vi "Disabled - Get File Names (SubVI).vi"(4 "Alliance Color Input":string, 5 "Reload File Names":bool, 6 "Running on Robot":bool=TRUE, 7 "Robot Path":string="/c/tmp/auton/", 8 "Computer Path":string="C:\\Users\\Pulsar\\Desktop\\FIRST 2012\\Autonomous\\1718 Read Auton Files\\") -> (0 "Alliance Color":string, 1 "Files Reloaded":bool, 2 "error out":errorcluster, 3 "File Name Array":string[](array[string]))   [LabVIEW 2020]
panel:
  in  "Change Alliance":bool
  in  "Message Delay (s)":dbl=1.0
  out "Number of Files":i32
  # "Inputs"
  # "Controls"
  # "Outputs"
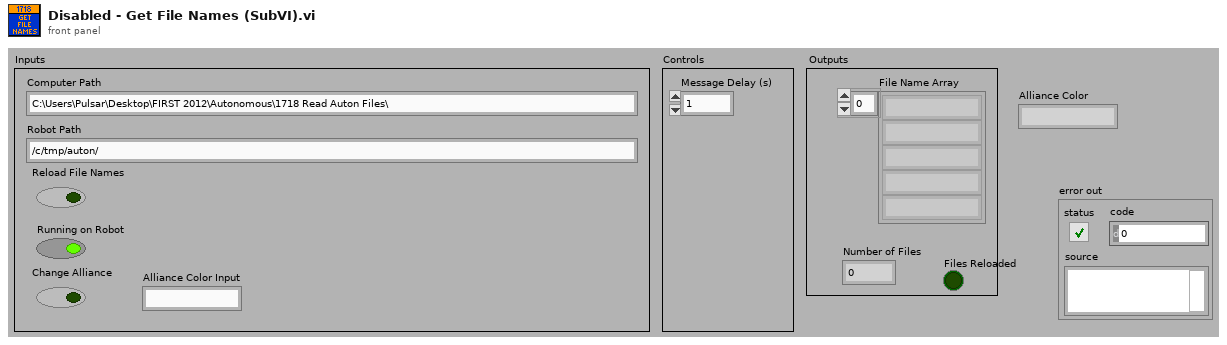
[diagram p1: front panel]
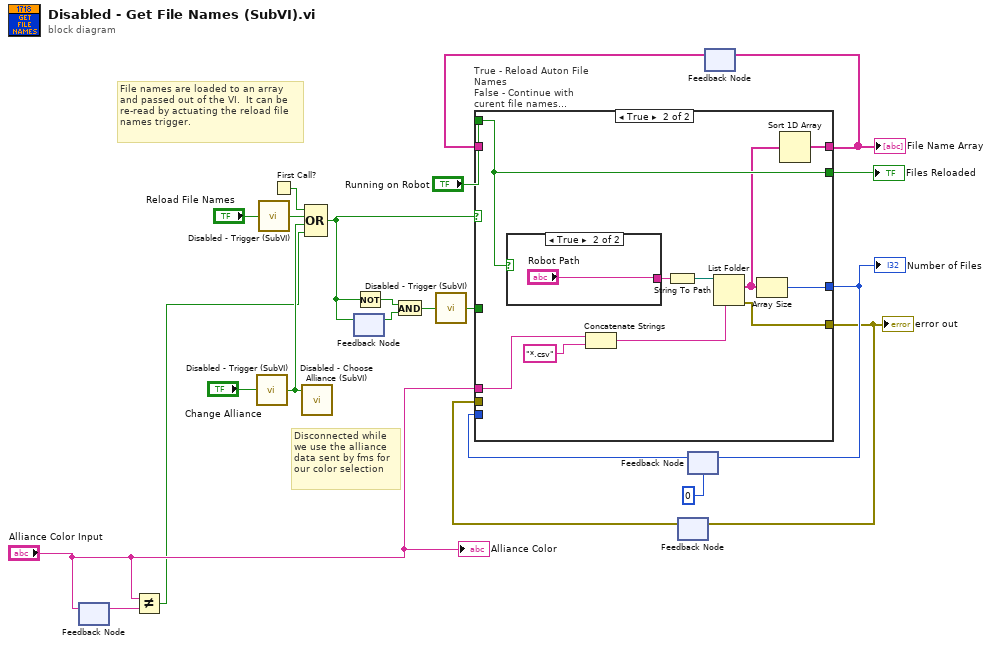
[diagram p0: block diagram]
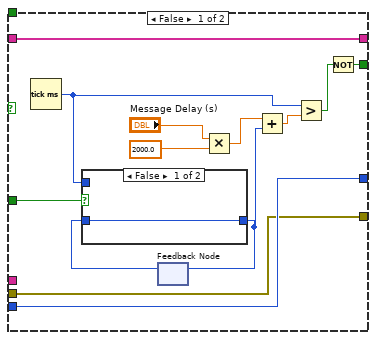
[diagram p2: hidden frame]
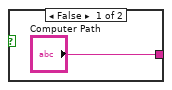
[diagram p4: hidden frame]
diagram:
  # "Disconnected while\nwe use the alliance\ndata sent by fms for\nour color selection"
  # "File names are loaded to an array\nand passed out of the VI.  It can be\nre-read by actuating the reload file\nnames trigger."
  n1 = feedback-in #1("Alliance Color Input") -> ()
  n2 = feedback #1() -> (w3:string)  [unwired: 1 in]
  n3 = Not Equal?(x="Alliance Color Input", y=w3) -> (x != y?=w1:bool)
  n4 = call "Disabled - Trigger (SubVI).vi"("Trigger"="Change Alliance") -> ("Trigger Output"=w12:bool)
  n5 = call "Disabled - Trigger (SubVI).vi"("Trigger"="Reload File Names") -> ("Trigger Output"=w13:bool)
  n6 = First Call?() -> (First Call?: T/F=w14:bool)
  n7 = call "Disabled - Choose Alliance (SubVI).vi"("Change Color"=w12) -> ()  [unwired: 10 in, 1 out]
  n8 = Compound Arithmetic op=OR(w14, w13, w12, w1) -> (w6:bool)
  n9 = feedback-in #2(w6) -> ()
  n10 = feedback #2() -> (w7:bool)  [unwired: 1 in]
  n11 = Not(x=w6) -> (.not. x?=w5:bool)
  n12 = And(x=w5, y=w7) -> (x .and. y?=w4:bool)
  n13 = call "Disabled - Trigger (SubVI).vi"("Trigger"=w4) -> ("Trigger Output"=w8:bool)
  n14 = feedback #3() -> (w9:errorcluster)  [unwired: 1 in]
  n15 = feedback #4(0) -> (w19:i32)
  n16 = feedback #5() -> (w21:string[])  [unwired: 1 out]
  n17 = case "True - Reload Auton File Names\nFalse - Continue with curent file names (loaded at startup)" shown="True" w6 {
    tunnel: [w35 w42] -> w22
    tunnel: [w34 w47] -> w20
    tunnel: w21 -> [w35 _]
    tunnel: w19 -> [w34 _]
    tunnel: "Running on Robot" -> [_ w44]
    tunnel: [w26 w44] -> w11
    tunnel: "Alliance Color Input" -> [_ w40]
    tunnel: [w24 w38] -> w10
    tunnel: w9 -> [w24 _]
    tunnel: w8 -> [w23 _]
    frame False {
      n18 = Tick Count (ms)() -> (millisecond timer value=w33:u32)
      n19 = feedback #6() -> (w32:u32)  [unwired: 1 in]
      n20 = case shown="False" w23 {
        tunnel: [w36 w37] -> w27
        tunnel: w33 -> [_ w37]
        tunnel: w32 -> [w36 _]
        frame False {
        }
        frame True {
        }
      }
      n21 = feedback-in #6(w27) -> ()
      n22 = Multiply(x="Message Delay (s)", y=2000.0) -> (x*y=w28:dbl)
      n23 = Add(x=w28, y=w27) -> (x+y=w31:dbl)
      n24 = Greater?(x=w33, y=w31) -> (0:w25:bool)
      n25 = Not(x=w25) -> (.not. x?=w26:bool)
    }
    frame True {
      n26 = case shown="True" w44 {
        tunnel: ["Computer Path" "Robot Path"] -> w45
        frame False {
        }
        frame True {
        }
      }
      n27 = Concatenate Strings(w40, "*.csv" ("pattern")) -> (w39:string)
      n28 = String To Path(string=w45) -> (path=w46:path)
      n29 = List Folder(path=w46, pattern=w39) -> (filenames=w43:string[], error out=w38:errorcluster)  [unwired: 1 in, 3 out]
      n30 = Array Size(array=w43) -> (size(s)=w47:i32)
      n31 = Sort 1D Array(array=w43) -> (sorted array=w42:string[])
    }
  }
  "File Name Array" <- w22
  "Number of Files" <- w20
  "Files Reloaded" <- w11
  "error out" <- w10
  n32 = feedback-in #3(w10) -> ()
  n33 = feedback-in #4(w20) -> ()
  n34 = feedback-in #5(w22) -> ()
  "Alliance Color" <- "Alliance Color Input"
